vi "Specific Path to Common Path.vi"(4 "specific path":path) -> (1 "common path":string)   [LabVIEW 2009]
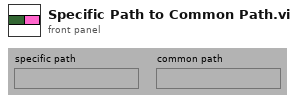
[diagram p1: front panel]
types:
  T1 = enum32{"invalid OS target", "Mac OS", "Windows 3.1", "Windows 95/NT", "Solaris 1", "Solaris 2", "HP-UX", "PowerMAX", "Linux", "Irix", "Rhapsody", "BeOS", "AIX", "OSF1", "VxWorks", "PharLap", "Carbon", "RTX", "Windows x64", "Linux x64"}
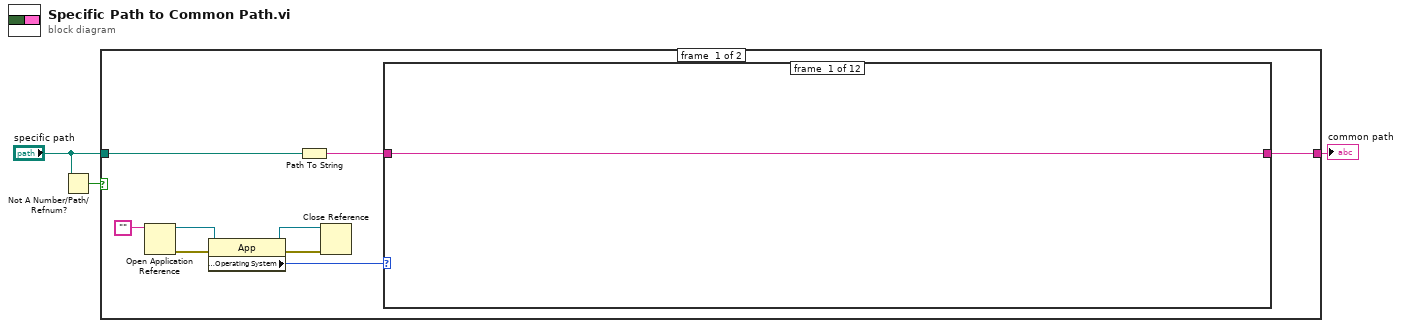
[diagram p0: block diagram]
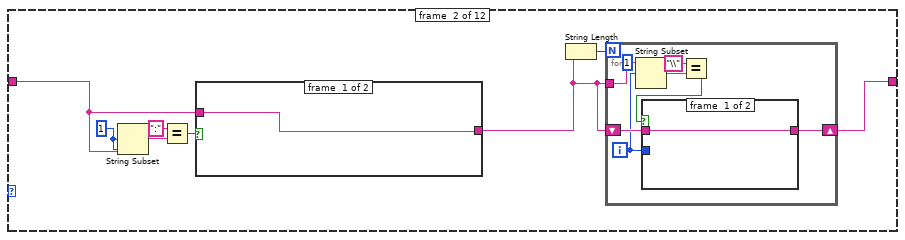
[diagram p2: hidden frame]
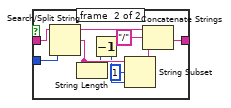
[diagram p3: hidden frame]
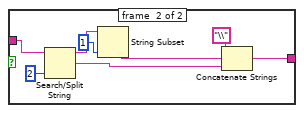
[diagram p4: hidden frame]
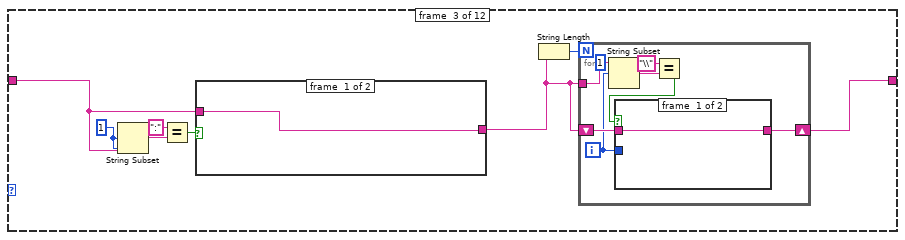
[diagram p5: hidden frame]
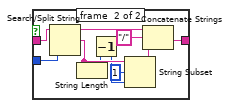
[diagram p6: hidden frame]
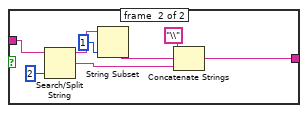
[diagram p7: hidden frame]
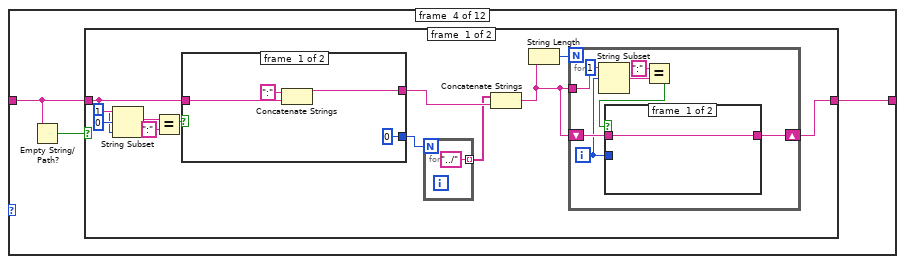
[diagram p8: hidden frame]
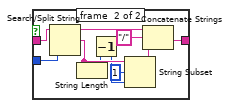
[diagram p9: hidden frame]
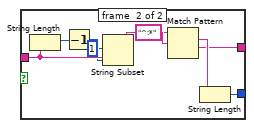
[diagram p10: hidden frame]
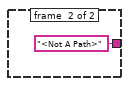
[diagram p20: hidden frame]
diagram:
  n1 = Not A Number/Path/Refnum?(number/path/refnum="specific path") -> (NaN/Path/Refnum?=w1:bool)
  n2 = case shown="False" w1 {
    tunnel: "specific path" -> [w12 _]
    tunnel: [w11 "<Not A Path>" ("string")] -> w3
    frame #0 {
      n3 = Open Application Reference(11:"") -> (0:w10:errorcluster, 3:w9:refnum<vi>)  [unwired: 3 in]
      n4 = property class="App"(reference=w9, error in=w10) -> (reference out=w7:refnum<vi>, error out=w8:errorcluster, "Application:Target:Operating System"=w4:T1)
      n5 = Path To String(path=w12) -> (string=w5:string)
      n6 = Close Reference(reference=w7, error in (no error)=w8) -> ()  [unwired: 1 out]
      n7 = case shown="\"Mac OS\", \"Carbon\"" w4 {
        tunnel: [w13 w14 w50 w88 w135 w136 w137 w138 w139 w140 w141 w142] -> w11
        tunnel: w5 -> [w13 w17 w53 w86 w135 w136 w137 w138 w139 w140 w141 w142]
        frame #0 {
        }
        frame #1 {
          w18 = 1 ("length")
          n8 = String Subset(string=w17, offset (0)=w18, length (rest)=w18) -> (substring=w21:string)
          n9 = Equal?(x=":", y=w21) -> (x = y?=w19:bool)
          n10 = case shown="True" w19 {
            tunnel: w17 -> [w41 w49]
            tunnel: [w41 w45] -> w15
            frame #0 {
            }
            frame #1 {
              n11 = Search/Split String(string=w49, offset (0)=2) -> (substring before match=w47:string, match + rest of string=w46:string)  [unwired: 1 in, 1 out]
              n12 = String Subset(string=w47, length (rest)=1 ("offset (0)")) -> (substring=w43:string)  [unwired: 1 in]
              n13 = Concatenate Strings("\\", w43, w46) -> (w45:string)
            }
          }
          n14 = String Length(string=w15) -> (length=w16:i32)
          n15 = for {
            N: w16 -> [_]
            tunnel: w15 -> [w27]
            shift-right: [w28] -> w14
            shift-left: w15 -> [w29]
            i -> [w26]
            n16 = String Subset(string=w27, offset (0)=w26, length (rest)=1 ("length")) -> (substring=w24:string)
            n17 = Equal?(x="\\", y=w24) -> (x = y?=w22:bool)
            n18 = case shown="True" w22 {
              tunnel: w29 -> [w30 w40]
              tunnel: w26 -> [_ w31]
              tunnel: [w30 w38] -> w28
              frame #0 {
              }
              frame #1 {
                n19 = Search/Split String(string=w40, offset (0)=w31) -> (substring before match=w39:string, match + rest of string=w36:string)  [unwired: 1 in, 1 out]
                n20 = String Length(string=w36) -> (length=w35:i32)
                n21 = Decrement(x=w35) -> (x-1=w34:i32)
                n22 = String Subset(string=w36, offset (0)=1, length (rest)=w34) -> (substring=w32:string)
                n23 = Concatenate Strings(w39, "/" ("x"), w32) -> (w38:string)
              }
            }
          }
        }
        frame #2 {
          w54 = 1 ("length")
          n24 = String Subset(string=w53, offset (0)=w54, length (rest)=w54) -> (substring=w57:string)
          n25 = Equal?(x=":", y=w57) -> (x = y?=w55:bool)
          n26 = case shown="True" w55 {
            tunnel: w53 -> [w77 w85]
            tunnel: [w77 w81] -> w51
            frame #0 {
            }
            frame #1 {
              n27 = Search/Split String(string=w85, offset (0)=2) -> (substring before match=w83:string, match + rest of string=w82:string)  [unwired: 1 in, 1 out]
              n28 = String Subset(string=w83, length (rest)=1 ("offset (0)")) -> (substring=w79:string)  [unwired: 1 in]
              n29 = Concatenate Strings("\\", w79, w82) -> (w81:string)
            }
          }
          n30 = String Length(string=w51) -> (length=w52:i32)
          n31 = for {
            N: w52 -> [_]
            tunnel: w51 -> [w63]
            shift-right: [w64] -> w50
            shift-left: w51 -> [w65]
            i -> [w62]
            n32 = String Subset(string=w63, offset (0)=w62, length (rest)=1 ("length")) -> (substring=w60:string)
            n33 = Equal?(x="\\", y=w60) -> (x = y?=w58:bool)
            n34 = case shown="True" w58 {
              tunnel: w65 -> [w66 w76]
              tunnel: w62 -> [_ w67]
              tunnel: [w66 w74] -> w64
              frame #0 {
              }
              frame #1 {
                n35 = Search/Split String(string=w76, offset (0)=w67) -> (substring before match=w75:string, match + rest of string=w72:string)  [unwired: 1 in, 1 out]
                n36 = String Length(string=w72) -> (length=w71:i32)
                n37 = Decrement(x=w71) -> (x-1=w70:i32)
                n38 = String Subset(string=w72, offset (0)=1, length (rest)=w70) -> (substring=w68:string)
                n39 = Concatenate Strings(w75, "/" ("x"), w68) -> (w74:string)
              }
            }
          }
        }
        frame #3 {
          n40 = Empty String/Path?(string/path=w86) -> (empty?=w87:bool)
          n41 = case shown="False" w87 {
            tunnel: w86 -> [w100 w134]
            tunnel: [w89 w134] -> w88
            frame #0 {
              n42 = String Subset(string=w100, offset (0)=0, length (rest)=1 ("length")) -> (substring=w97:string)
              n43 = Equal?(x=w97, y=":") -> (x = y?=w95:bool)
              n44 = case shown="False" w95 {
                tunnel: w100 -> [w124 w133]
                tunnel: [w122 w127] -> w93
                tunnel: [0 w126] -> w94
                frame #0 {
                  n45 = Concatenate Strings(":", w124) -> (w122:string)
                }
                frame #1 {
                  n46 = String Length(string=w133) -> (length=w132:i32)
                  n47 = Decrement(x=w132) -> (x-1=w131:i32)
                  n48 = String Subset(string=w133, offset (0)=1 ("length"), length (rest)=w131) -> (substring=w125:string)
                  n49 = Match Pattern(string=w125, regular expression="^:*") -> (match substring=w128:string, after substring=w127:string)  [unwired: 1 in, 2 out]
                  n50 = String Length(string=w128) -> (length=w126:i32)
                }
              }
              n51 = for {
                N: w94 -> [_]
                tunnel: ["../"] -> w92 mode=indexing
              }
              n52 = Concatenate Strings(w92, w93) -> (w90:string)
              n53 = String Length(string=w90) -> (length=w91:i32)
              n54 = for {
                N: w91 -> [_]
                tunnel: w90 -> [w106]
                shift-right: [w107] -> w89
                shift-left: w90 -> [w108]
                i -> [w105]
                n55 = String Subset(string=w106, offset (0)=w105, length (rest)=1 ("length")) -> (substring=w103:string)
                n56 = Equal?(x=":", y=w103) -> (x = y?=w101:bool)
                n57 = case shown="True" w101 {
                  tunnel: w108 -> [w109 w119]
                  tunnel: w105 -> [_ w110]
                  tunnel: [w109 w117] -> w107
                  frame #0 {
                  }
                  frame #1 {
                    n58 = Search/Split String(string=w119, offset (0)=w110) -> (substring before match=w118:string, match + rest of string=w115:string)  [unwired: 1 in, 1 out]
                    n59 = String Length(string=w115) -> (length=w114:i32)
                    n60 = Decrement(x=w114) -> (x-1=w113:i32)
                    n61 = String Subset(string=w115, offset (0)=1, length (rest)=w113) -> (substring=w111:string)
                    n62 = Concatenate Strings(w118, "/" ("x"), w111) -> (w117:string)
                  }
                }
              }
            }
            frame #1 {
            }
          }
        }
        frame #4 {
        }
        frame #5 {
        }
        frame #6 {
        }
        frame #7 {
        }
        frame #8 {
        }
        frame #9 {
        }
        frame #10 {
        }
        frame #11 {
        }
      }
    }
    frame #1 {
    }
  }
  "common path" <- w3
